vi "Load Xml.vi"(8 "error in":errorcluster caption="错误输入（无错误）", 10 "selected path":path caption="所选路径", 11 "PanelRootNode 输入":refnum<class "PanelRootNode.lvclass"> caption="DNL_LabVIEW Object in") -> (0 "error out":errorcluster caption="错误输出", 3 "PanelRootNode 输出":refnum<class "PanelRootNode.lvclass"> caption="DNL_LabVIEW Object out")   [LabVIEW 2013, in "PanelRootNode.lvclass"]
uses:
  PanelRootNode.lvclass
  <vilib>/xml/Load XML File.vi
  <vilib>/xml/Close Reference(Node).vi
  <vilib>/xml/NI_XML.lvlib
  <resource>/objmgr/DOMUserDefRef.rc
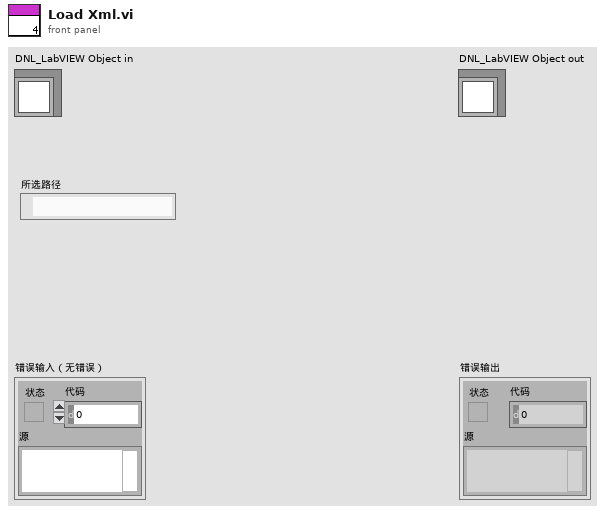
[diagram p1: front panel]
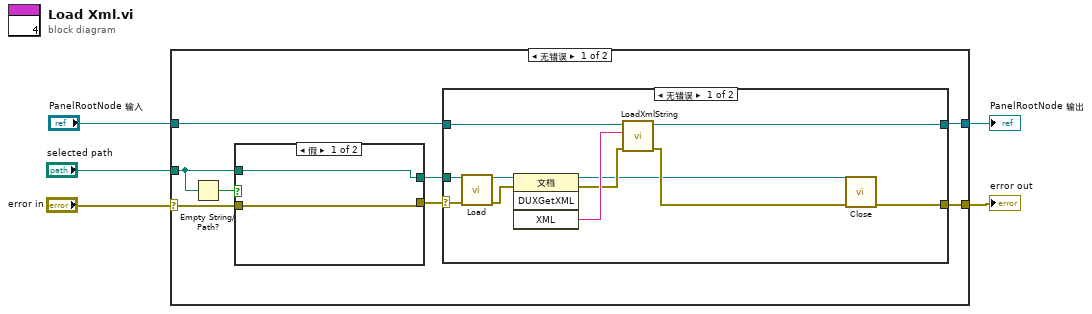
[diagram p0: block diagram]
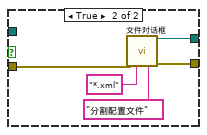
[diagram p2: hidden frame]
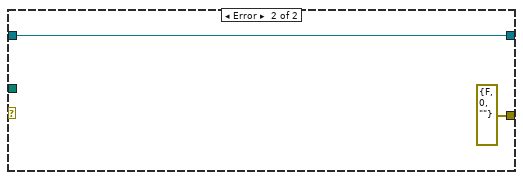
[diagram p3: hidden frame]
diagram:
  n1 = case shown="无错误" "error in" {
    selector: "error in" -> [w9 w35]
    tunnel: [w10 w35] -> w4
    tunnel: [w13 w34] -> w2
    tunnel: "PanelRootNode 输入" -> [w6 w34]
    tunnel: "selected path" -> [w7 _]
    frame No Error {
      n2 = Empty String/Path?(string/path=w7) -> (empty?=w8:bool)
      n3 = case shown="假" w8 {
        tunnel: [w15 w20] -> w12
        tunnel: [w14 w19] -> w11
        tunnel: w9 -> [w14 w18]
        tunnel: w7 -> [w15 _]
        frame False {
        }
        frame True {
          n4 = call "文件对话框"("error in"=w18, "pattern (all files)"="*.xml", "pattern label"="分割配置文件") -> ("selected path"=w20:path, "error out"=w19:errorcluster)  [unwired: 9 in, 2 out]
        }
      }
      n5 = case shown="无错误" w11 {
        selector: w11 -> [w30 _]
        tunnel: w6 -> [w29 w33]
        tunnel: [w28 w33] -> w13
        tunnel: w12 -> [w31 _]
        tunnel: [w26 errorcluster {"status"=FALSE, "code"=0, "source"=""} ("error out")] -> w10
        frame No Error {
          n6 = call-poly <vilib>:"Load.vi"("path to XML document"=w31, "error in (no error)"=w30) -> ("DOM document out"=w25:refnum<k20>, "error out"=w23:errorcluster)  [unwired: 11 in, 1 out]
          n7 = invoke class="文档" method="DUXGetXML"(reference=w25, error in=w23) -> (reference out=w21:refnum<k20>, error out=w22:errorcluster, "XML"=w24:string)  [unwired: 2 in, 1 out]
          n8 = call-dynamic "LoadXmlString.vi"("error in"=w22, "XmlString"=w24, "PanelRootNode 输入"=w29) -> ("error out"=w27:errorcluster, "PanelRootNode 输出"=w28:refnum<class "PanelRootNode.lvclass">)  [unwired: 7 in]
          n9 = call-poly <vilib>:"Close.vi"("error in (no error)"=w27, "node"=w21) -> ("error out"=w26:errorcluster)  [unwired: 7 in]
        }
        frame Error {
        }
      }
    }
    frame Error {
    }
  }
  "error out" <- w4
  "PanelRootNode 输出" <- w2
